vi "Build Object ID List.vi"(8 "error in":errorcluster, 11 "object layouts":refnum<class "Object Layout.lvclass">[](array[class])) -> (0 "error out":errorcluster, 3 "object ID list":variant)   [LabVIEW 2010, in "NI_SE_Front Panel Layout.lvlib"]
uses:
  NI_SE_Front Panel Layout.lvlib
  Object Layout Classes/Object Layout/Object Layout.lvclass
  Object Layout Classes/Object Layout/Object Layout.lvclass/Object Layout.ctl
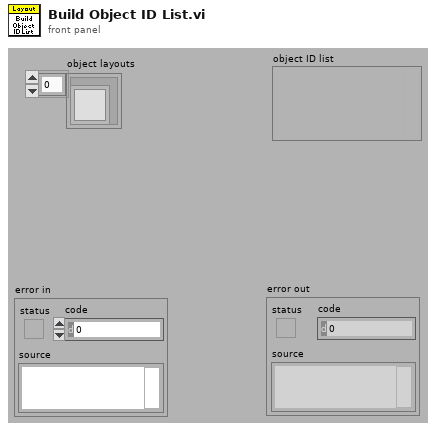
[diagram p1: front panel]
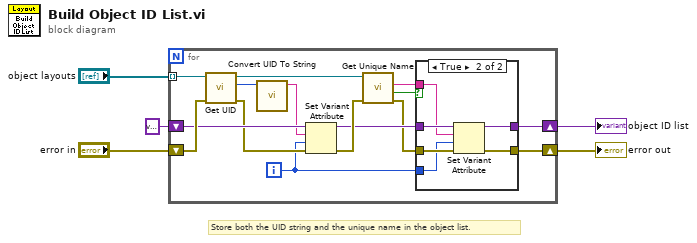
[diagram p0: block diagram]
diagram:
  # "Store both the UID string and the unique name in the object list."
  n1 = for {
    tunnel: "object layouts" -> [w20] mode=indexing
    shift-right: [w9] -> w1
    shift-left: "error in" -> [w19]
    shift-right: [w11] -> w2
    shift-left: variant -> [w18]
    i -> [w7]
    n2 = call "Get UID.vi"("error in (no error)"=w19, "Object Layout in"=w20) -> ("error out"=w17:errorcluster, "UID"=w14:i32, "Object Layout out"=w16:refnum<class "Object Layout.lvclass">)  [unwired: 7 in]
    n3 = call "Convert UID To String.vi"("UID"=w14) -> ("UID string"=w13:string)  [unwired: 10 in]
    n4 = Set Variant Attribute(Variant=w18, name=w13, value=w7, error in=w17) -> (Variant out=w12:variant, error out=w15:errorcluster)  [unwired: 1 out]
    n5 = call "Get Unique Name.vi"("error in (no error)"=w15, "Object Layout in"=w16) -> ("error out"=w10:errorcluster, "found?"=w6:bool, "unique name"=w8:string)  [unwired: 6 in, 1 out]
    n6 = case shown="True" w6 {
      tunnel: w12 -> [w22 w28]
      tunnel: [w22 w27] -> w11
      tunnel: w10 -> [w21 w26]
      tunnel: [w21 w25] -> w9
      tunnel: w8 -> [_ w24]
      tunnel: w7 -> [_ w23]
      frame False {
      }
      frame True {
        n7 = Set Variant Attribute(Variant=w28, name=w24, value=w23, error in=w26) -> (Variant out=w27:variant, error out=w25:errorcluster)  [unwired: 1 out]
      }
    }
  }
  "error out" <- w1
  "object ID list" <- w2
